vi "Configure Internal Trigger.vi"(8 "error in (no error)":errorcluster, 10 "Internal Trigger Rate (1 MHz)":dbl, 11 "DG645 in":refnum<class "DG645.lvclass">) -> (0 "error out":errorcluster, 3 "DG645 out":refnum<class "DG645.lvclass">)   [LabVIEW 2018, in "DG645.lvlib" / "DG645.lvclass"]
uses:
  DG645.lvclass
  DG645.lvclass/DG645.ctl
  <instrlib>/Stanford Research DG645/Stanford Research DG645.lvlib
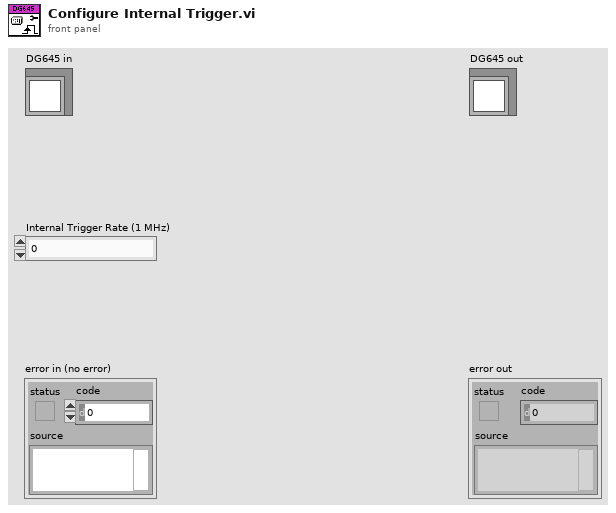
[diagram p1: front panel]
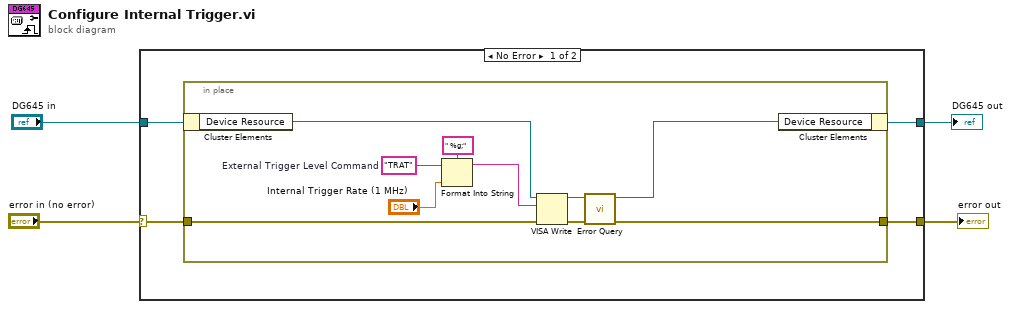
[diagram p0: block diagram]
diagram:
  n1 = case shown="No Error" "error in (no error)" {
    selector: "error in (no error)" -> [w7 w19]
    tunnel: "DG645 in" -> [w8 w20]
    tunnel: [w6 w19] -> w2
    tunnel: [w5 w20] -> w1
    frame No Error {
      n2 = in-place {
        in-place-border: w7 -> [w11]
        in-place-border: [w12] -> w6
        w14 = "TRAT"  # External Trigger Level Command
        n3 = in-place-cluster #1(w8) -> ("Device Resource"=w9:refnum<visa-resource-name>)
        n4 = Format Into String(format string=" %g;" ("Source Command"), initial string=w14, "Internal Trigger Rate (1 MHz)") -> (resulting string=w16:string)  [unwired: 1 in, 1 out]
        n5 = VISA Write(VISA resource name=w9, write buffer=w16, error in (no error)=w11) -> (VISA resource name out=w18:refnum<visa-resource-name>, error out=w17:errorcluster)  [unwired: 1 out]
        n6 = call <instrlib>:"Error Query.vi"("error in (no error)"=w17, "VISA resource name"=w18) -> ("error out"=w12:errorcluster, "VISA resource name out"=w13:refnum<visa-resource-name>)  [unwired: 6 in, 2 out]
        n7 = in-place-cluster #1("Device Resource"=w13) -> (w5:refnum<class "DG645.lvclass">)
      }
    }
    frame Error {
    }
  }
  "error out" <- w2
  "DG645 out" <- w1
